vi "Tegam4040_Set_Global.vi"(8 "Tegam2_DAC_Offset_100V":dbl, 9 "Tegam1_DAC_Offset_100V":dbl, 10 "Tegam2_DAC_Offset_10V":dbl, 11 "Tegam1_DAC_Offset_10V":dbl) -> ()   [LabVIEW 2010]
uses:
  Tegam4040_Offset_Global.vi
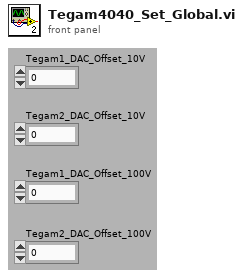
[diagram p1: front panel]
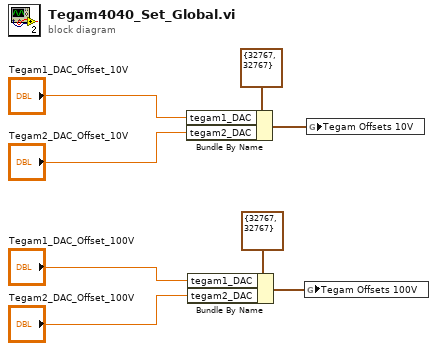
[diagram p0: block diagram]
diagram:
  n1 = Bundle By Name(cluster=cluster{"tegam2_DAC":u16, "tegam1_DAC":u16} {"tegam2_DAC"=32767, "tegam1_DAC"=32767} ("Tegam Offsets"), "tegam1_DAC"="Tegam1_DAC_Offset_10V", "tegam2_DAC"="Tegam2_DAC_Offset_10V") -> (w7:cluster{"tegam2_DAC":u16, "tegam1_DAC":u16})
  n2 = Bundle By Name(cluster=cluster{"tegam2_DAC":u16, "tegam1_DAC":u16} {"tegam2_DAC"=32767, "tegam1_DAC"=32767} ("Tegam Offsets"), "tegam1_DAC"="Tegam1_DAC_Offset_100V", "tegam2_DAC"="Tegam2_DAC_Offset_100V") -> (w3:cluster{"tegam2_DAC":u16, "tegam1_DAC":u16})
  n3 = global write "Tegam4040_Offset_Global.vi" "Tegam Offsets 100V"(w3) -> ()
  n4 = global write "Tegam4040_Offset_Global.vi" "Tegam Offsets 10V"(w7) -> ()
